vi "Server.vi"() -> ()   [LabVIEW 2015]
uses:
  <vilib>/Platform/TimedLoop/XDataNode/timing_clust.ctl
  <vilib>/Platform/TimedLoop/XDataNode/nitl_modes.ctl
  <vilib>/Platform/TimedLoop/XDataNode/wakeup.ctl
  <vilib>/platform/TimedLoop/XDataNode/XDataNode.xnode
  <vilib>/Platform/TimedLoop/XDataNode/XDNodeRunTimeDep.lvlib
panel:
  out "output cluster":T1
  out "Time":u32
  out "Tries":u32
  out "Average Delay (ms)":dbl
  out "Delay (ms)":u32
  in  "stop":bool
  # "Overview:  Coding that exemplifies how to benchmark the communication of Shared Variables.\nRequirements: LabVIEW 2012 or compatible\nInstructions:\n1.  Run the \"Benchmark SV Receive LV2012 - NI Verified.vi\"\n2. Run this VI\n3. Watch the amount of time it takes to communicate\n4. Stop both VIs"
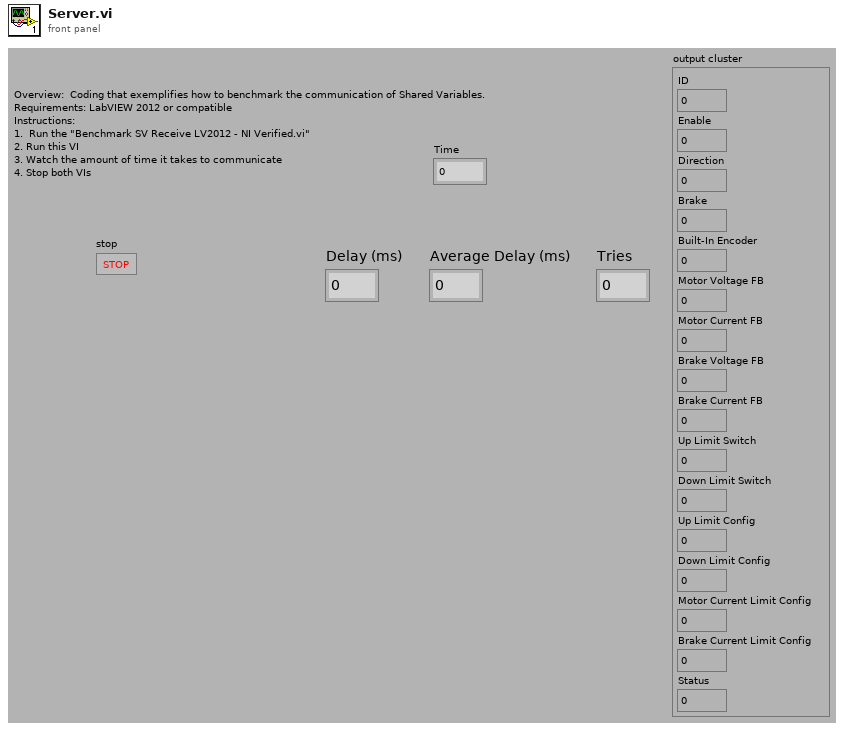
[diagram p1: front panel]
types:
  T1 = cluster{"ID":dbl, "Enable":dbl, "Direction":dbl, "Brake":dbl, "Built-In Encoder":dbl, "Motor Voltage FB":dbl, "Motor Current FB":dbl, "Brake Voltage FB":dbl, "Brake Current FB":dbl, "Up Limit Switch":dbl, "Down Limit Switch":dbl, "Up Limit Config":dbl, "Down Limit Config":dbl, "Motor Current Limit Config":dbl, "Brake Current Limit Config":dbl, "Status":dbl}
  T2 = typedef "XDNodeRunTimeDep.lvlib/timing_clust.ctl" = cluster{"Expected End [f-1]":u64, "Actual End [f-1]":u64, "Finished Late? [f-1]":bool, "Expected End [i-1]":u64, "Actual End [i-1]":u64, "Finished Late? [i-1]":bool, "Expected Start [i]":u64, "Actual Start [i]":u64, "Expected Start [f]":u64, "Actual Start [f]":u64, "Source Name":string, "Structure Name":string, "Period":i64, "Deadline":i64, "Offset":i64, "Start":i64, "Priority":i32, "Timeout":i32, "Mode":T3, "Wakeup Reason":T4, "Error":errorcluster, "Source Type":string, "Secondary Source Type":string, "Global End Time":u64, "Global Start Time":u64, "Frame Duration":u64, "Iteration Duration":u64, "Assigned CPU":i32, "I/O Scan Engine Mode":u32}
  T3 = typedef "XDNodeRunTimeDep.lvlib/nitl_modes.ctl" = enum32{"No Change", "Process missed periods, maintain original phase", "Discard missed periods, maintain original phase", "Process missed periods, ignore original phase", "Discard missed periods, ignore original phase"}
  T4 = typedef "XDNodeRunTimeDep.lvlib/wakeup.ctl" = enum32{"Normal", "Aborted", "Asynchronous wakeup", "Timing source error", "Timed loop error", "Timeout"}
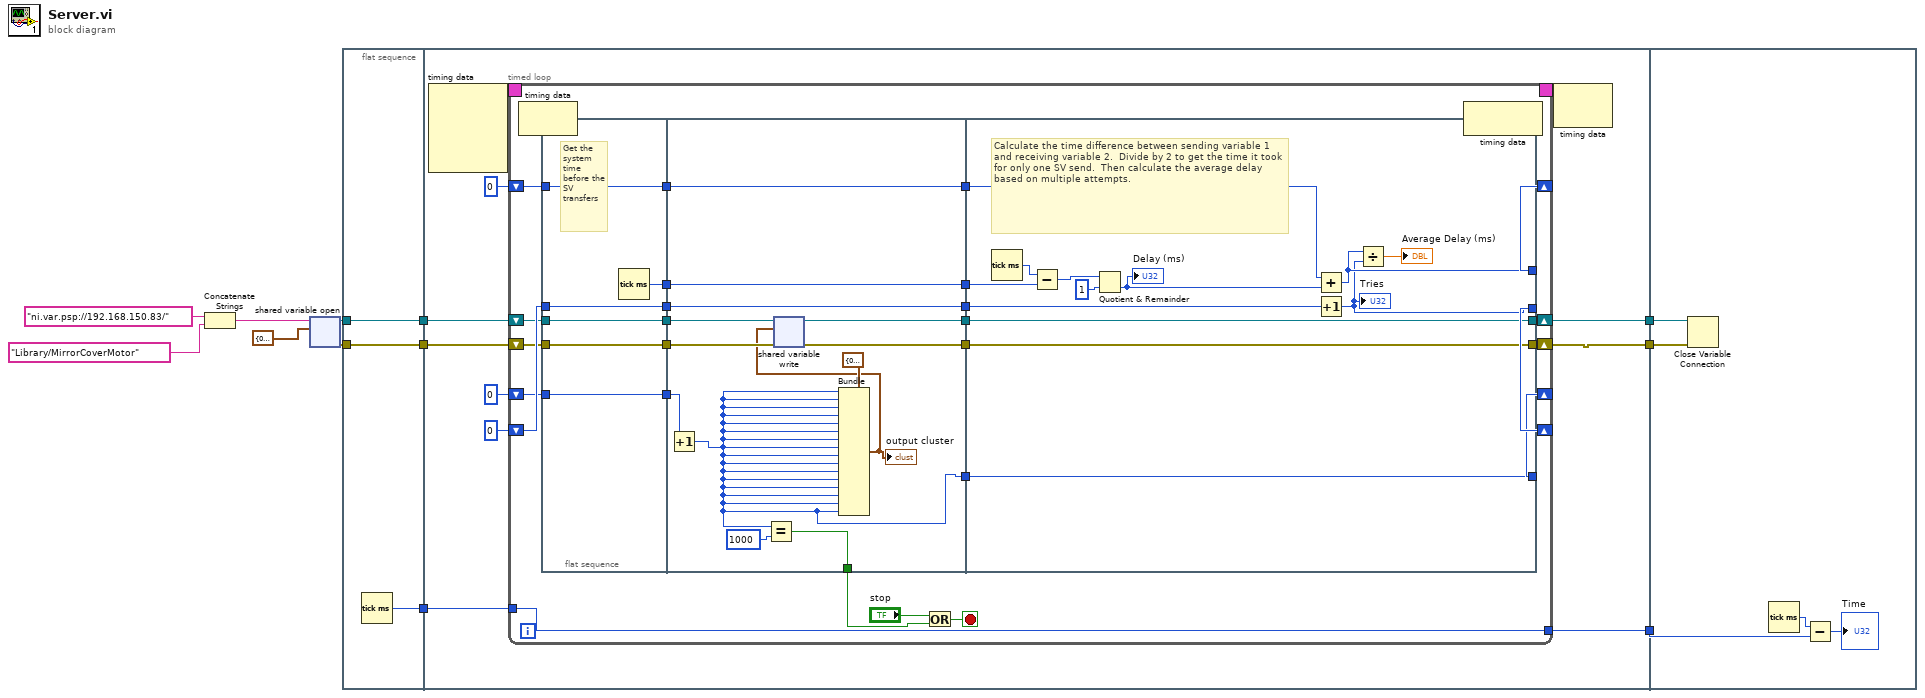
[diagram p0: block diagram]
diagram:
  n1 = Concatenate Strings("ni.var.psp://192.168.150.83/" ("string"), "Library/MirrorCoverMotor") -> (w12:string)
  n2 = shared-variable-open(w12, T1 {"ID"=0.0, "Enable"=0.0, "Direction"=0.0, "Brake"=0.0, "Built-In Encoder"=0.0, "Motor Voltage FB"=0.0, "Motor Current FB"=0.0, "Brake Voltage FB"=0.0, "Brake Current FB"=0.0, "Up Limit Switch"=0.0, "Down Limit Switch"=0.0, "Up Limit Config"=0.0, "Down Limit Config"=0.0, "Motor Current Limit Config"=0.0, "Brake Current Limit Config"=0.0, "Status"=0.0} ("MirrorCoverMotor")) -> (w10:refnum<k21>, w11:errorcluster)  [unwired: 2 in]
  n3 = flat-sequence {
    tunnel: w10 -> [w14]
    tunnel: w11 -> [w15]
    tunnel: [w15] -> w6
    tunnel: [w14] -> w5
    tunnel: [w13] -> w4
    tunnel: [w21] -> w7
    tunnel: w6 -> [w23]
    tunnel: w5 -> [w22]
    tunnel: w4 -> [w20]
    tunnel: [w19] -> w3
    tunnel: [w18] -> w2
    tunnel: w7 -> [w91]
    tunnel: w3 -> [w90]
    tunnel: w2 -> [w89]
    frame #0 {
      n4 = Tick Count (ms)() -> (millisecond timer value=w13:u32)
    }
    frame #1 {
      n5 = node-c288() -> (w17:T2)  [unwired: 4 in]
      n6 = timed-loop {
        shift-right: [w52] -> _
        shift-left: u32 0 -> [w46]
        shift-right: [w51] -> _
        shift-left: u32 0 -> [w47]
        shift-right: [w43] -> _
        shift-left: u64 0 -> [w44]
        shift-right: [w35] -> w19
        shift-left: w23 -> [w33]
        shift-right: [w30] -> w18
        shift-left: w22 -> [w28]
        tunnel: [w27] -> w21
        tunnel: w20 -> [w27]
        timing: w17 -> [_]
        timing-out: [_] -> w16
        stop <- w42 stop-if-true
        n7 = node-c288() -> ()  [unwired: 1 in, 1 out]
        n8 = flat-sequence {
          tunnel: [w58] -> w50
          tunnel: [w60] -> w49
          tunnel: [w59] -> w48
          tunnel: [w57] -> w45
          tunnel: [w56] -> w32
          tunnel: [w55] -> w31
          tunnel: w46 -> [w60]
          tunnel: w47 -> [w59]
          tunnel: w44 -> [w57]
          tunnel: w33 -> [w56]
          tunnel: w28 -> [w55]
          tunnel: [w73] -> w39
          tunnel: [w72] -> w38
          tunnel: [w71] -> w37
          tunnel: w50 -> [w73]
          tunnel: w49 -> [w72]
          tunnel: w48 -> [w71]
          tunnel: w45 -> [w63]
          tunnel: [w61] -> w36
          tunnel: [w69] -> w40
          tunnel: [w68] -> w34
          tunnel: w32 -> [w67]
          tunnel: w31 -> [w66]
          tunnel: [w65] -> w29
          tunnel: w39 -> [w85]
          tunnel: [w78] -> w52
          tunnel: w38 -> [w80]
          tunnel: [w77] -> w51
          tunnel: w37 -> [w84]
          tunnel: w36 -> [w76]
          tunnel: [w76] -> w43
          tunnel: [w75] -> w35
          tunnel: w34 -> [w75]
          tunnel: [w74] -> w30
          tunnel: w29 -> [w74]
          frame #0 {
            # "Get the system time before the SV transfers"
            n9 = Tick Count (ms)() -> (millisecond timer value=w58:u32)
          }
          frame #1 {
            n10 = Increment(x=w63) -> (x+1=w61:u64)
            n11 = Equal?(x=w61, y=u64 1000) -> (x = y?=w69:bool)
            n12 = Bundle(cluster=T1 {"ID"=0.0, "Enable"=0.0, "Direction"=0.0, "Brake"=0.0, "Built-In Encoder"=0.0, "Motor Voltage FB"=0.0, "Motor Current FB"=0.0, "Brake Voltage FB"=0.0, "Brake Current FB"=0.0, "Up Limit Switch"=0.0, "Down Limit Switch"=0.0, "Up Limit Config"=0.0, "Down Limit Config"=0.0, "Motor Current Limit Config"=0.0, "Brake Current Limit Config"=0.0, "Status"=0.0} ("MirrorCoverMotor"), "ID"=w61, "Enable"=w61, "Direction"=w61, "Brake"=w61, "Built-In Encoder"=w61, "Motor Voltage FB"=w61, "Motor Current FB"=w61, "Brake Voltage FB"=w61, "Brake Current FB"=w61, "Up Limit Switch"=w61, "Down Limit Switch"=w61, "Up Limit Config"=w61, "Down Limit Config"=w61, "Motor Current Limit Config"=w61, "Brake Current Limit Config"=w61, "Status"=w61) -> (w62:T1)
            "output cluster" <- w62
            n13 = shared-variable-write(w66, w67, w62) -> (w65:refnum<k21>, w68:errorcluster)
          }
          frame #2 {
            # "Calculate the time difference between sending variable 1 and receiving variable 2.  Divide by 2 to get the time it took for only one SV send.  Then calculate the average delay based on multiple attempts."
            n14 = Tick Count (ms)() -> (millisecond timer value=w86:u32)
            n15 = Subtract(x=w86, y=w85) -> (x-y=w83:u32)
            n16 = Quotient & Remainder(x=w83, y=u32 1) -> (floor(x/y)=w81:u32)  [unwired: 1 out]
            "Delay (ms)" <- w81
            n17 = Add(x=w80, y=w81) -> (x+y=w78:u32)
            n18 = Increment(x=w84) -> (x+1=w77:u32)
            "Tries" <- w77
            n19 = Divide(x=w78, y=w77) -> (x/y=→"Average Delay (ms)":dbl)
          }
        }
        n20 = Or(x="stop", y=w40) -> (x .or. y?=w42:bool)
        n21 = node-c288() -> ()  [unwired: 1 in, 1 out]
      }
      n22 = node-c288(w16) -> ()  [unwired: 1 out]
    }
    frame #2 {
      n23 = Close Variable Connection(8:w90, 11:w89) -> ()  [unwired: 1 out]
      n24 = Tick Count (ms)() -> (millisecond timer value=w93:u32)
      n25 = Subtract(x=w93, y=w91) -> (x-y=→"Time":u32)
    }
  }
